vi "CH_LM Config Analog Output Full Scale Voltage.vi"(0 "Meter Index":i32, 2 "Analog Out \nFullscale Voltage (2V)":T1=enum."2 V", 5 "error in (no error)":errorcluster, 7 "Timeout / ms (3000)":i32=3000, 8 "Action (query)":bool, 9 "Lock Timeout / ms (1000)":i32=1000) -> (11 "Lock timed out":bool, 14 "Meter Index":i32, 16 "Analog Out \nFullscale Voltage":T1=enum."2 V", 19 "error out":errorcluster)   [LabVIEW 2012, in "CH_LM.lvlib"]
doc: "This command will set/query the full scale output voltage at the analog output connector."
uses:
  CH_LM.lvlib
  CH_LM AnalogOutFullscaleVoltage.ctl
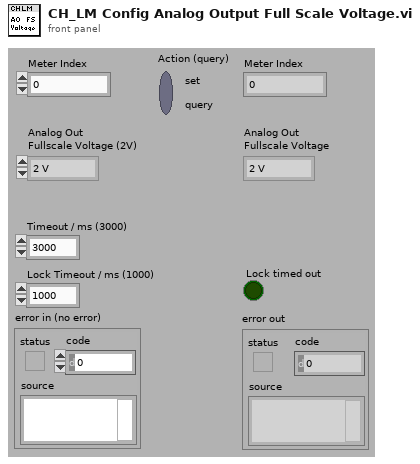
[diagram p1: front panel]
types:
  T1 = typedef "CH_LM.lvlib/CH_LM AnalogOutFullscaleVoltage.ctl" = enum16{"1 V", "2 V", "4 V"}
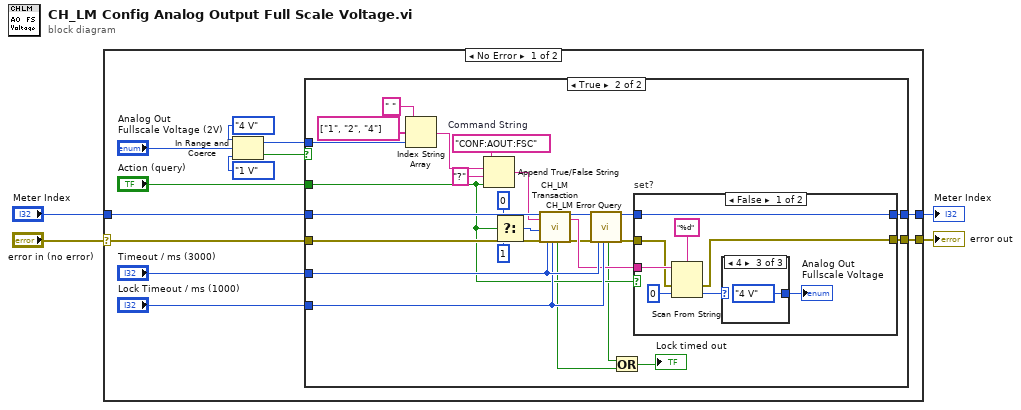
[diagram p0: block diagram]
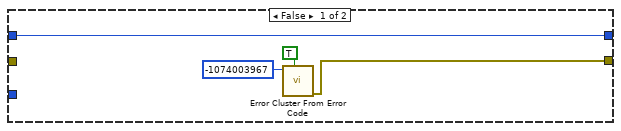
[diagram p2: hidden frame]
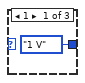
[diagram p3: hidden frame]
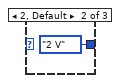
[diagram p4: hidden frame]
diagram:
  n1 = case shown="No Error" "error in (no error)" {
    selector: "error in (no error)" -> [w16 w60]
    tunnel: [w14 w60] -> w4
    tunnel: "Meter Index" -> [w15 w59]
    tunnel: [w13 w59] -> w1
    frame No Error {
      n2 = In Range and Coerce(upper limit=CH_LM_AnalogOutFullscaleVoltage."4 V" ("Analog Out \nFullscale Voltage (2V)"), x="Analog Out \nFullscale Voltage (2V)", lower limit=CH_LM_AnalogOutFullscaleVoltage."1 V" ("Analog Out \nFullscale Voltage (2V)")) -> (coerced(x)=w9:T1, In Range?=w7:bool)
      n3 = case shown="True" w7 {
        tunnel: w16 -> [_ w45]
        tunnel: w15 -> [w20 w44]
        tunnel: [w17 w43] -> w14
        tunnel: [w20 w42] -> w13
        tunnel: "Timeout / ms (3000)" -> [_ w41]
        tunnel: "Lock Timeout / ms (1000)" -> [_ w40]
        tunnel: "Action (query)" -> [_ w39]
        tunnel: w9 -> [_ w25]
        frame False {
          n4 = call <vilib>:"Error Cluster From Error Code.vi"("show call chain? (False)"=TRUE, "error code (0)"=-1074003967) -> ("error out"=w17:errorcluster)  [unwired: 1 in, 6 out]
        }
        frame True {
          w38 = "CONF:AOUT:FSC"  # Command String
          n5 = Index String Array(1:w25, 2:string[] ["1", "2", "4"] ("string array"), 3:" ") -> (0:w22:string)
          n6 = Append True/False String(1:w39, 2:"?" ("true string"), 3:w22, 4:w38) -> (0:w21:string)
          n7 = Select(t=0, s=w39, f=1 ("NofStrings (-1:all)")) -> (s? t:f=w34:i32)
          n8 = call "CH_LM Transaction.vi"("Meter Index"=w44, "Command String"=w21, "NofStrings (-1:all)"=w34, "error in (no error)"=w45, "Timeout / ms (3000)"=w41, "Lock Timeout / ms (1000)"=w40) -> ("Lock timed out"=w27:bool, "Meter Index"=w32:i32, "Response"=w37:string, "error out"=w30:errorcluster)  [unwired: 10 out]
          n9 = call "CH_LM Error Query.vi"("Meter Index"=w32, "error in (no error)"=w30, "Timeout / ms (3000)"=w41, "Lock Timeout / ms (1000)"=w40) -> ("Lock timed out"=w28:bool, "Meter Index"=w31:i32, "error out"=w29:errorcluster)  [unwired: 13 out]
          n10 = Or(x=w28, y=w27) -> (x .or. y?=→"Lock timed out":bool)
          n11 = case "set?" shown="False" w39 {
            tunnel: w37 -> [w53 _]
            tunnel: w29 -> [w52 w58]
            tunnel: [w51 w58] -> w43
            tunnel: w31 -> [w48 w57]
            tunnel: [w48 w57] -> w42
            frame False {
              n12 = Scan From String(format string="%d", input string=w53, error in=w52, default 1=u16 0 ("default value 1")) -> (error out=w51:errorcluster, output 1=w47:u16)  [unwired: 1 in, 2 out]
              n13 = case shown="4" w47 {
                tunnel: [CH_LM_AnalogOutFullscaleVoltage."1 V" ("Analog Out \nFullscale Voltage") CH_LM_AnalogOutFullscaleVoltage."2 V" ("Analog Out \nFullscale Voltage") CH_LM_AnalogOutFullscaleVoltage."4 V" ("Analog Out \nFullscale Voltage")] -> w46
                frame 1 {
                }
                frame 2, Default {
                }
                frame 4 {
                }
              }
              "Analog Out \nFullscale Voltage" <- w46
            }
            frame True {
            }
          }
        }
      }
    }
    frame Error {
    }
  }
  "error out" <- w4
  "Meter Index" <- w1
